vi "非国标启动命令.vi"(7 "参数下拉列表":u16(ring) items=["总磷"=1, "总氮"=2], 8 "Error in":errorcluster caption="Error in (no error)", 9 "量程下拉列表":enum16{"低量程", "高量程"}(ring), 10 "测量模式":T1(ring), 11 "MB session in":refnum<class "MB_Master.lvclass">) -> (0 "error out":errorcluster, 3 "MB session out":refnum<class "MB_Master.lvclass">)   [LabVIEW 2016, in "斯坦道总磷.lvlib"]
uses:
  <vilib>/Plasmionique/MB Master/MB_Master/MB_Master.lvclass
  <vilib>/Plasmionique/MB Master/MB Master.lvlib
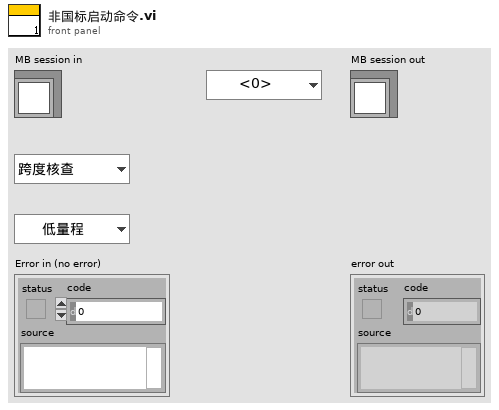
[diagram p1: front panel]
types:
  T1 = enum16{"跨度核查", "水样测量", "零点核查", "标样核查", "加标回收", "快捷测试", "空白校准", "标样校准"}
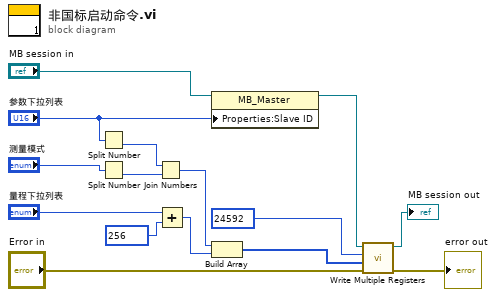
[diagram p0: block diagram]
diagram:
  n1 = Split Number(x="参数下拉列表") -> (lo(x)=w7:u8)  [unwired: 1 out]
  n2 = Split Number(x="测量模式") -> (lo(x)=w8:u8)  [unwired: 1 out]
  n3 = Join Numbers(hi=w7, lo=w8) -> ((hi.lo)=w6:u16)
  n4 = Add(x="量程下拉列表", y=u16 256 ("starting address")) -> (x+y=w2:u16)
  n5 = property class="MB_Master"(reference="MB session in", "Properties:Slave ID"="参数下拉列表") -> (reference out=w10:refnum<class "MB_Master.lvclass">)  [unwired: 1 in, 1 out]
  n6 = Build Array(w6, w2) -> (w5:u16[])
  n7 = call <vilib>:"Write Multiple Registers.vi"("error in (no error)"="Error in", "values"=w5, "starting address"=u16 24592, "MB session in"=w10) -> ("error out"=→"error out":errorcluster, "MB session out"=→"MB session out":refnum<class "MB_Master.lvclass">)  [unwired: 6 in]
